vi "Add Alarm.vi"(8 "error in (no error)":errorcluster, 11 "Alarm":errorcluster) -> (0 "error out":errorcluster)   [LabVIEW 2020, in "Alarms Handler Actor API.lvclass"]
uses:
  Alarms Handler Actor API.lvclass
  Base Actor/API/Actor API.lvclass/Actor API.ctl
  C:/dev/PGS/2001 - TBCM/Source/RT/RTAF/Source/RTAF/Actors/Base Actor/API/Actor API.lvclass
  RTAF Global References.vi
  Base Actor/API/Actor API.lvclass
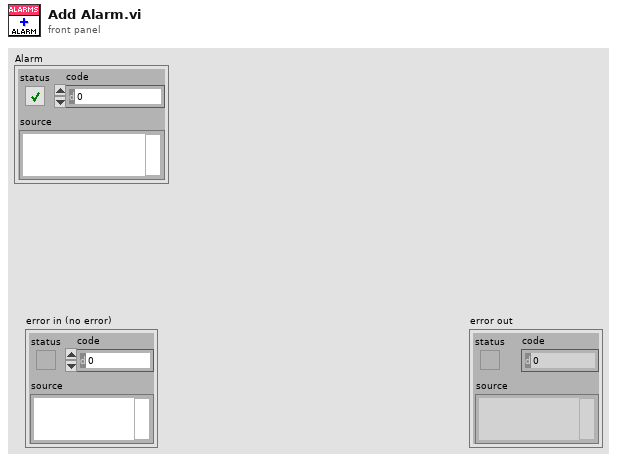
[diagram p1: front panel]
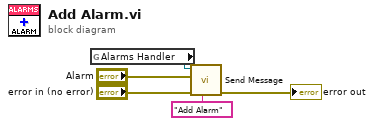
[diagram p0: block diagram]
diagram:
  n1 = global read "RTAF Global References.vi" "Alarms Handler"() -> (w1:refnum<class "Alarms Handler Actor API.lvclass">)
  n2 = call "Send Message.vi"("Name"="Add Alarm", "error in (no error)"="error in (no error)", "Payload"="Alarm", "Actor API in"=w1) -> ("error out"=→"error out":errorcluster)  [unwired: 7 in]
